vi "MatchCutTime.vi"(5 "Default End Time (0)":dbl, 7 "Default Start Time (0)":dbl, 10 "Keyword Matching":T1(array[cluster]), 11 "Filename":string) -> (2 "End Time":dbl, 3 "Start Time":dbl)   [LabVIEW 2015]
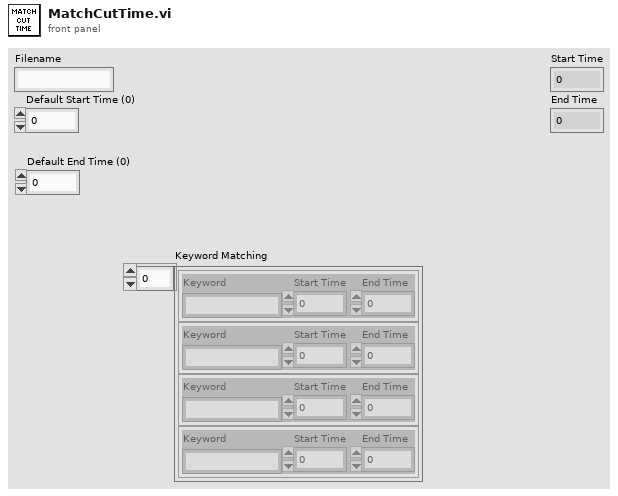
[diagram p1: front panel]
types:
  T1 = cluster{"Keyword":string, "Start Time":dbl, "End Time":dbl}[]
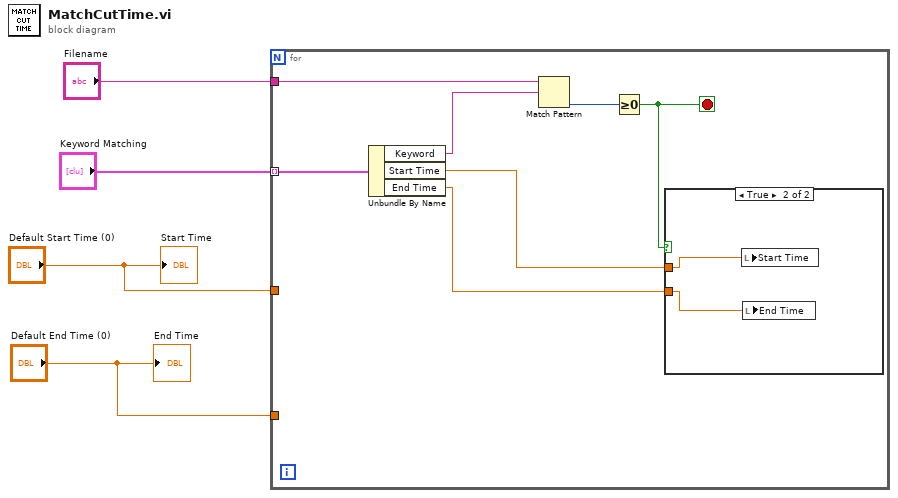
[diagram p0: block diagram]
diagram:
  n1 = for {
    tunnel: "Keyword Matching" -> [w11] mode=indexing
    tunnel: "Filename" -> [w10]
    tunnel: "Default Start Time (0)" -> [_]
    tunnel: "Default End Time (0)" -> [_]
    stop <- w7 stop-if-true
    n2 = Unbundle By Name(w11) -> ("Keyword"=w9:string, "Start Time"=w6:dbl, "End Time"=w5:dbl)
    n3 = Match Pattern(string=w10, regular expression=w9) -> (offset past match=w8:i32)  [unwired: 1 in, 3 out]
    n4 = Greater Or Equal To 0?(x=w8) -> (x >= 0?=w7:bool)
    n5 = case shown="True" w7 {
      tunnel: w6 -> [_ w13]
      tunnel: w5 -> [_ w12]
      frame False {
      }
      frame True {
        n6 = local write "Start Time"(w13) -> ()
        n7 = local write "End Time"(w12) -> ()
      }
    }
  }
  "Start Time" <- "Default Start Time (0)"
  "End Time" <- "Default End Time (0)"
